vi "DisplayExecution Event Callback.vi"(4 "User Parameter":T1, 5 "Event data":cluster{"exec":refnum<k7>, "reason":i32}, 6 "CtlRef":refnum<k7>, 7 "Event common data":cluster{"Source":i32, "Type":u32, "Time":u32}) -> ()   [LabVIEW 2010, in "TS Simple LabVIEW OI Dependencies.lvlib"]
uses:
  TS Simple LabVIEW OI Dependencies.lvlib
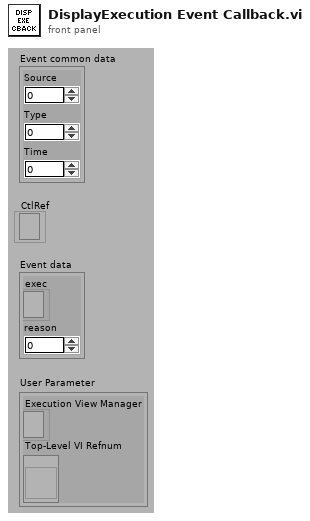
[diagram p1: front panel]
types:
  T1 = cluster{"Execution View Manager":refnum<k7>, "Top-Level VI Refnum":refnum<vi>}
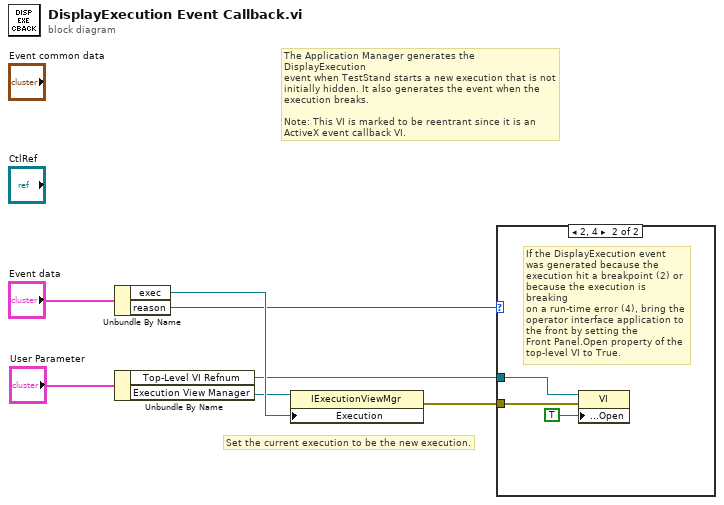
[diagram p0: block diagram]
diagram:
  # "The Application Manager generates the DisplayExecution\nevent when TestStand starts a new execution that is not\ninitially hidden. It also generates the event when the\nexecution breaks.\n\nNote: This VI is marked to be reentrant since it is an\nActiveX event callback VI."
  # "Set the current execution to be the new execution."
  n1 = Unbundle By Name("Event data") -> ("exec"=w7:refnum<k7>, "reason"=w5:i32)
  n2 = Unbundle By Name("User Parameter") -> ("Top-Level VI Refnum"=w1:refnum<vi>, "Execution View Manager"=w2:refnum<k7>)
  n3 = property class="IExecutionViewMgr"(reference=w2, "Execution"=w7) -> (error out=w4:errorcluster)  [unwired: 1 in, 1 out]
  n4 = case shown="2, 4" w5 {
    tunnel: w4 -> [_ w10]
    tunnel: w1 -> [_ w9]
    frame Default {
    }
    frame 2, 4 {
      # "If the DisplayExecution event\nwas generated because the\nexecution hit a breakpoint (2) or\nbecause the execution is breaking\non a run-time error (4), bring the\noperator interface application to\nthe front by setting the\nFront Panel.Open property of the\ntop-level VI to True."
      n5 = property class="VI"(reference=w9, error in=w10, "Front Panel Window:Open"=TRUE) -> ()  [unwired: 2 out]
    }
  }
